vi "_Get Bookmarks.vi"(8 "error in (no error)":errorcluster, 9 "show vi in llb?":bool, 11 "App Info":T1) -> (0 "error out":errorcluster, 2 "possible undisplayed bookmarks":bool, 3 "bookmarks":T2[](array[typedef]))   [LabVIEW 2017, in "CSM_ExampleBrowser.lvlib"]
uses:
  CSM_ExampleBrowser.lvlib
  controls/BMark_Bookmark Data.ctl
  controls/BMark_VI_Identifier.ctl
  <vilib>/addons/analyzer/_analyzerctrls.llb/VIAnCtl Analysis App Info.ctl
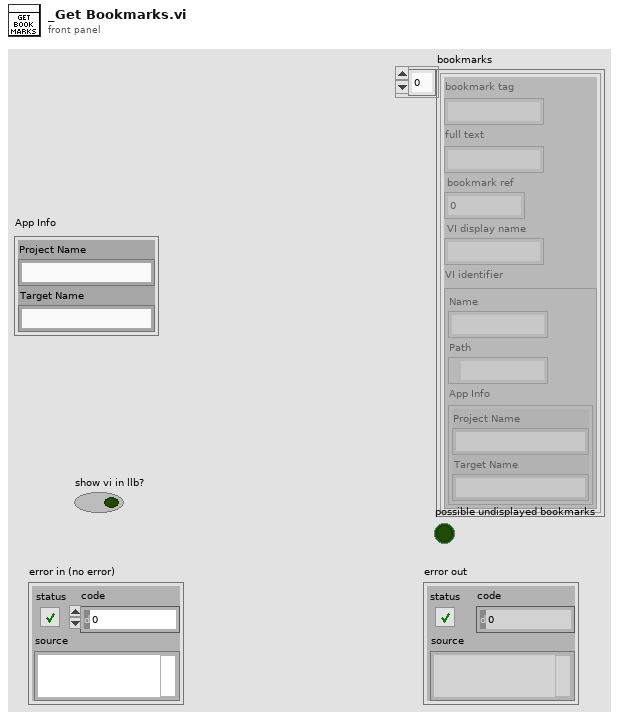
[diagram p1: front panel]
types:
  T1 = typedef "VIAnCtl Analysis App Info.ctl" = cluster{"Project Name":string, "Target Name":string}
  T2 = typedef "CSM_ExampleBrowser.lvlib/BMark_Bookmark Data.ctl" = cluster{"bookmark tag":string, "full text":string, "bookmark ref":i32, "VI display name":string, "VI identifier":T3}
  T3 = typedef "CSM_ExampleBrowser.lvlib/BMark_VI_Identifier.ctl" = cluster{"Name":string, "Path":path, "App Info":T1}
  T4 = typedef "CSM_ExampleBrowser.lvlib/BMark_Array of Bookmarks.ctl" = T5[]
  T5 = typedef "CSM_ExampleBrowser.lvlib/BMark_Bookmark Cluster.ctl" = cluster{"bookmark ref":i32, "bookmark":string, "label text":string, "VI identifier":T3}
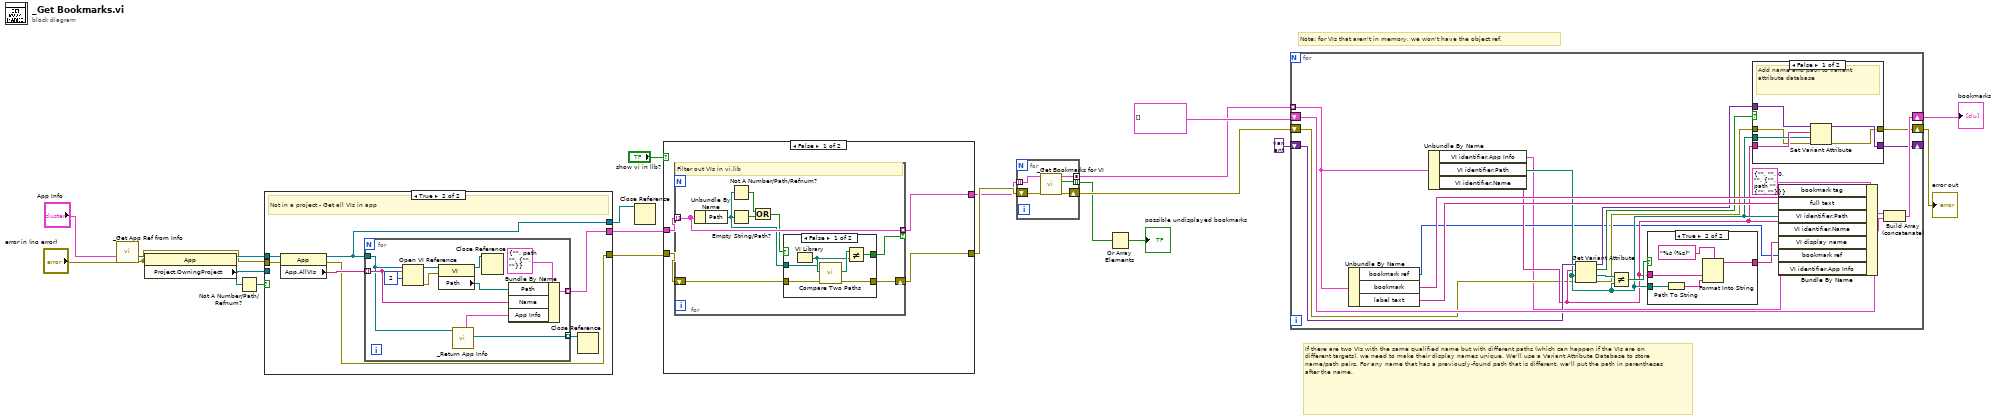
[diagram p0: block diagram]
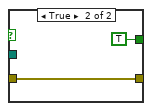
[diagram p2: hidden frame]
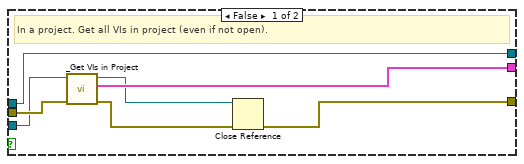
[diagram p4: hidden frame]
diagram:
  # "Note: for VIs that aren't in memory, we won't have the object ref."
  # "If there are two VIs with the same qualified name but with different paths (which can happen if the VIs are on different targets), we need to make their display names unique. We'll use a Variant Attribute Database to store name/path pairs. For any name that has a previously-found path that is different, we'll put the path in parentheses after the name."
  n1 = call "_Get App Ref from Info.vi"("error in (no error)"="error in (no error)", "Analysis App Info"="App Info") -> ("error out"=w3:errorcluster, "Analysis App ref"=w5:refnum<vi>)  [unwired: 8 in]
  n2 = property class="App"(reference=w5, error in=w3) -> (reference out=w18:refnum<vi>, "Project.OwningProject"=w17:refnum<vi>)  [unwired: 1 out]
  n3 = Not A Number/Path/Refnum?(number/path/refnum=w17) -> (NaN/Path/Refnum?=w19:bool)
  n4 = case shown="True" w19 {
    tunnel: w18 -> [w26 w35]
    tunnel: w17 -> [w24 _]
    tunnel: [w22 w31] -> w13
    tunnel: w3 -> [w28 w34]
    tunnel: [w27 w32] -> w11
    tunnel: [w26 w30] -> w2
    frame False {
      # "In a project. Get all VIs in project (even if not open)."
      n5 = call "_Get VIs in Project.vi"("error in (no error)"=w28, "project"=w24) -> ("error out"=w25:errorcluster, "Array of VIs"=w27:T3[], "project out"=w23:refnum<vi>)  [unwired: 7 in]
      n6 = Close Reference(reference=w23, error in (no error)=w25) -> (error out=w22:errorcluster)
    }
    frame True {
      # "Not in a project - Get all VIs in app"
      n7 = property class="App"(reference=w35, error in=w34) -> (reference out=w30:refnum<vi>, error out=w31:errorcluster, "App.AllVIs"=w33:string[])
      n8 = for {
        tunnel: w33 -> [w41] mode=indexing
        tunnel: [w45] -> w32 mode=indexing
        tunnel: w30 -> [w40]
        tunnel: [w37] -> w29 mode=indexing
        n9 = Open VI Reference(application reference (local)=w40, vi path=w41, options=2) -> (vi reference=w44:refnum<vi>, error out=w43:errorcluster)  [unwired: 3 in]
        n10 = property class="VI"(reference=w44, error in=w43) -> (reference out=w38:refnum<vi>, "Path"=w42:path)  [unwired: 1 out]
        n11 = call "_Return App Info.vi"("App Refnum in"=w40) -> ("App Refnum for Opening VI"=w37:refnum<vi>, "App Info"=w39:T1)  [unwired: 8 in, 1 out]
        n12 = Close Reference(reference=w38) -> ()  [unwired: 1 in, 1 out]
        n13 = Bundle By Name(cluster=T3 {"Name"="", "Path"=path "", "App Info"={"Project Name"="", "Target Name"=""}} ("Cluster"), "Path"=w42, "Name"=w41, "App Info"=w39) -> (w45:T3)
      }
      n14 = Close Reference(reference=w29) -> ()  [unwired: 1 in, 1 out]
    }
  }
  n15 = Close Reference(reference=w2) -> ()  [unwired: 1 in, 1 out]
  n16 = case shown="False" "show vi in llb?" {
    tunnel: w13 -> [w50 w68]
    tunnel: [w48 w68] -> w12
    tunnel: w11 -> [w49 w67]
    tunnel: [w47 w67] -> w10
    frame False {
      n17 = for {
        shift-right: [w57] -> w48
        shift-left: w50 -> [w58]
        tunnel: w49 -> [w55] mode=indexing
        tunnel: [w55] -> w47 mode=indexing if=w56
        # "Filter out VIs in vi.lib"
        n18 = Unbundle By Name(w55) -> ("Path"=w54:path)
        n19 = Not A Number/Path/Refnum?(number/path/refnum=w54) -> (NaN/Path/Refnum?=w53:bool)
        n20 = Empty String/Path?(string/path=w54) -> (empty?=w52:bool)
        n21 = Or(x=w53, y=w52) -> (x .or. y?=w51:bool)
        n22 = case shown="False" w51 {
          tunnel: w58 -> [w62 w65]
          tunnel: [w61 w65] -> w57
          tunnel: w54 -> [w60 _]
          tunnel: [w59 TRUE] -> w56
          frame False {
            n23 = VI Library() -> (path=w63:path)
            n24 = call <vilib>:"Compare Two Paths.vi"("error in (no error)"=w62, "Path 2"=w63, "Path 1"=w60) -> ("error out"=w61:errorcluster, "Common Path"=w64:path)  [unwired: 5 in, 2 out]
            n25 = Not Equal?(x=w64, y=w63) -> (x != y?=w59:bool)
          }
          frame True {
          }
        }
      }
    }
    frame True {
    }
  }
  n26 = for {
    shift-right: [w72] -> w15
    shift-left: w12 -> [w73]
    tunnel: [w71] -> w16 mode=concatenating
    tunnel: w10 -> [w70] mode=indexing
    tunnel: [w69] -> w8 mode=indexing
    n27 = call "_Get Bookmarks for VI.vi"("error in (no error)"=w73, "VI"=w70) -> ("error out"=w72:errorcluster, "possible undisplayed bookmarks"=w69:bool, "Array of bookmarks"=w71:T4)  [unwired: 7 in]
  }
  n28 = Or Array Elements(Boolean array=w8) -> (logical OR=→"possible undisplayed bookmarks":bool)
  n29 = for {
    shift-right: [w93] -> w20
    shift-left: T2[] [] -> [w94]
    tunnel: w16 -> [w79] mode=indexing
    shift-right: [w80] -> w14
    shift-left: w15 -> [w76]
    shift-right: [w88] -> _
    shift-left: variant -> [w87]
    n30 = Unbundle By Name(w79) -> ("bookmark ref"=w75:i32, "bookmark"=w89:string, "label text"=w90:string)
    n31 = Unbundle By Name(w79) -> ("VI identifier.App Info"=w74:T1, "VI identifier.Path"=w78:path, "VI identifier.Name"=w77:string)
    n32 = Get Variant Attribute(Variant=w87, name=w77, default value (empty Variant)=w78, error in=w76) -> (duplicate Variant=w83:variant, found=w82:bool, value=w86:path, error out=w81:errorcluster)
    n33 = Not Equal?(x=w86, y=w78) -> (x != y?=w84:bool)
    n34 = case shown="True" w84 {
      tunnel: w78 -> [_ w106]
      tunnel: w77 -> [w103 w105]
      tunnel: [w103 w104] -> w85
      frame False {
      }
      frame True {
        n35 = Path To String(path=w106) -> (string=w107:string)
        n36 = Format Into String(format string="%s (%s)", w105, w107) -> (resulting string=w104:string)  [unwired: 2 in, 1 out]
      }
    }
    n37 = case shown="False" w82 {
      tunnel: [w100 w102] -> w88
      tunnel: w83 -> [w99 w102]
      tunnel: w77 -> [w98 _]
      tunnel: w78 -> [w97 _]
      tunnel: w81 -> [w96 w101]
      tunnel: [w95 w101] -> w80
      frame False {
        # "Add name and path to variant attribute database"
        n38 = Set Variant Attribute(Variant=w99, name=w98, value=w97, error in=w96) -> (Variant out=w100:variant, error out=w95:errorcluster)  [unwired: 1 out]
      }
      frame True {
      }
    }
    n39 = Bundle By Name(cluster=T2 {"bookmark tag"="", "full text"="", "bookmark ref"=0, "VI display name"="", "VI identifier"={"Name"="", "Path"=path "", "App Info"={"Project Name"="", "Target Name"=""}}} ("bookmark item"), "bookmark tag"=w89, "full text"=w90, "VI identifier.Path"=w78, "VI identifier.Name"=w77, "VI display name"=w85, "bookmark ref"=w75, "VI identifier.App Info"=w74) -> (w91:T2)
    n40 = Build Array (concatenate)(w94, w91) -> (w93:T2[])
  }
  "bookmarks" <- w20
  "error out" <- w14
